vi "activacion_fotosensores.vi"(5 "Cabina":dbl(slide) scale=1.0..5.0) -> (0 "In Range? 3":bool, 1 "In Range? 5":bool, 2 "In Range? 2":bool, 3 "In Range?":bool, 4 "In Range? 4":bool)   [LabVIEW 2021]
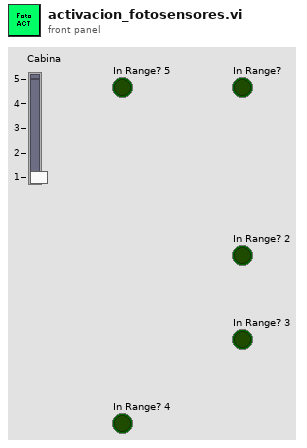
[diagram p1: front panel]
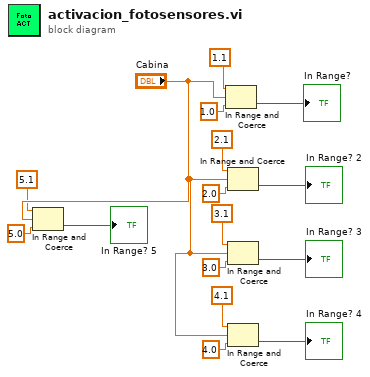
[diagram p0: block diagram]
diagram:
  n1 = In Range and Coerce(upper limit=5.1, x="Cabina", lower limit=5.0) -> (In Range?=→"In Range? 5":bool)  [unwired: 1 out]
  n2 = In Range and Coerce(upper limit=1.1, x="Cabina", lower limit=1.0) -> (In Range?=→"In Range?":bool)  [unwired: 1 out]
  n3 = In Range and Coerce(upper limit=2.1, x="Cabina", lower limit=2.0) -> (In Range?=→"In Range? 2":bool)  [unwired: 1 out]
  n4 = In Range and Coerce(upper limit=3.1, x="Cabina", lower limit=3.0) -> (In Range?=→"In Range? 3":bool)  [unwired: 1 out]
  n5 = In Range and Coerce(upper limit=4.1, x="Cabina", lower limit=4.0) -> (In Range?=→"In Range? 4":bool)  [unwired: 1 out]
